vi "scheduledEnable.vi"(2 "Scheduler on?":bool, 3 "Disable time":T1 {"minute" min=0 max=59 step=1; "hour" min=0 max=23 step=1}, 4 "Enable time":T1 {"minute" min=0 max=59 step=1; "hour" min=0 max=23 step=1}) -> (0 "Enable?":bool)   [LabVIEW 2017]
uses:
  Schedule time.ctl
panel:
  # ":"
  # ":"
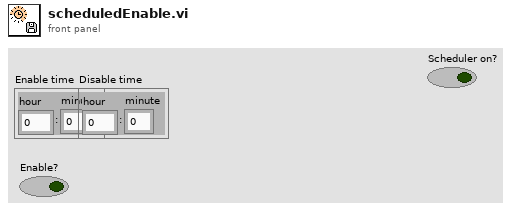
[diagram p1: front panel]
types:
  T1 = typedef "Schedule time.ctl" = cluster{"minute":i32, "hour":i32}
  T2 = typedef "LVDateTimeRec.ctl" = cluster{"fractional second":dbl, "second":i32, "minute":i32, "hour":i32, "day of month":i32, "month":i32, "year":i32, "day of week":i32, "day of year":i32, "DST":i32}
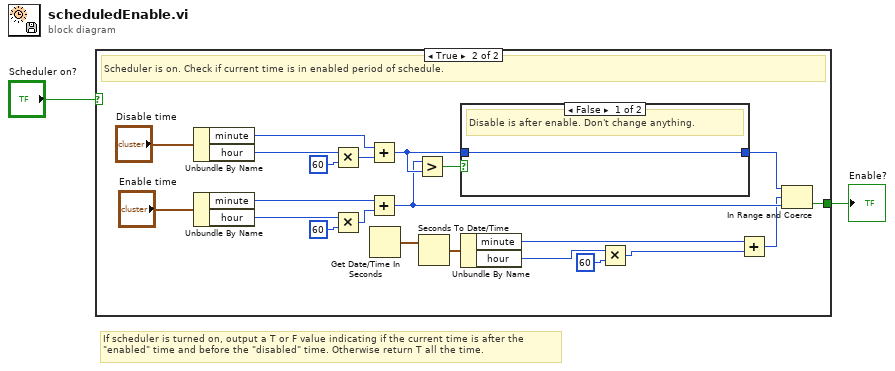
[diagram p0: block diagram]
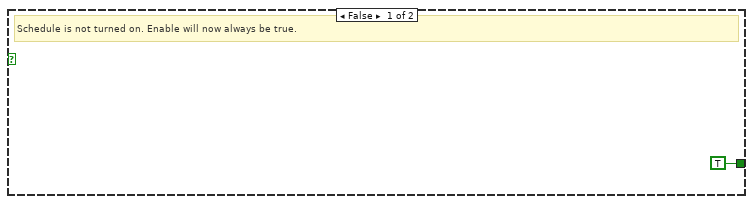
[diagram p2: hidden frame]
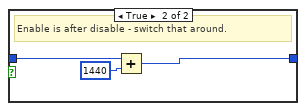
[diagram p3: hidden frame]
diagram:
  # "If scheduler is turned on, output a T or F value indicating if the current time is after the \n\"enabled\" time and before the \"disabled\" time. Otherwise return T all the time."
  n1 = case shown="True" "Scheduler on?" {
    tunnel: [TRUE w4] -> w1
    frame False {
      # "Schedule is not turned on. Enable will now always be true."
    }
    frame True {
      # "Scheduler is on. Check if current time is in enabled period of schedule."
      n2 = Unbundle By Name "Unbundle By Name"("Disable time") -> ("minute"=w11:i32, "hour"=w17:i32)
      n3 = Unbundle By Name "Unbundle By Name"("Enable time") -> ("minute"=w10:i32, "hour"=w18:i32)
      n4 = Multiply(x=w17, y=60 ("hour")) -> (x*y=w14:i32)
      n5 = Multiply(x=w18, y=60 ("hour")) -> (x*y=w15:i32)
      n6 = Add(x=w11, y=w14) -> (x+y=w8:i32)
      n7 = Add(x=w10, y=w15) -> (x+y=w7:i32)
      n8 = Get Date/Time In Seconds() -> (seconds since 1Jan1904=w24:timestamp)
      n9 = Greater?(x=w7, y=w8) -> (0:w9:bool)
      n10 = Seconds To Date/Time(time stamp (now)=w24) -> (date time rec=w23:T2)  [unwired: 1 in]
      n11 = case shown="False" w9 {
        tunnel: w8 -> [w26 w28]
        tunnel: [w26 w27] -> w6
        frame False {
          # "Disable is after enable. Don't change anything."
        }
        frame True {
          # "Enable is after disable - switch that around."
          n12 = Add(x=w28, y=1440 ("hour")) -> (x+y=w27:i32)
        }
      }
      n13 = Unbundle By Name "Unbundle By Name"(w23) -> ("minute"=w12:i32, "hour"=w16:i32)
      n14 = Multiply(x=w16, y=60 ("hour")) -> (x*y=w13:i32)
      n15 = Add(x=w12, y=w13) -> (x+y=w5:i32)
      n16 = In Range and Coerce(upper limit=w6, x=w5, lower limit=w7) -> (In Range?=w4:bool)  [unwired: 1 out]
    }
  }
  "Enable?" <- w1
